vi "Write Observation Title.vi"(8 "error in (no error)":errorcluster, 10 "OBS_TITLE.Value":string, 11 "Save Image in":refnum<class "Save Image.lvclass">) -> (0 "error out":errorcluster, 3 "Save Image out":refnum<class "Save Image.lvclass">)   [LabVIEW 2018]
uses:
  Save Image.lvclass
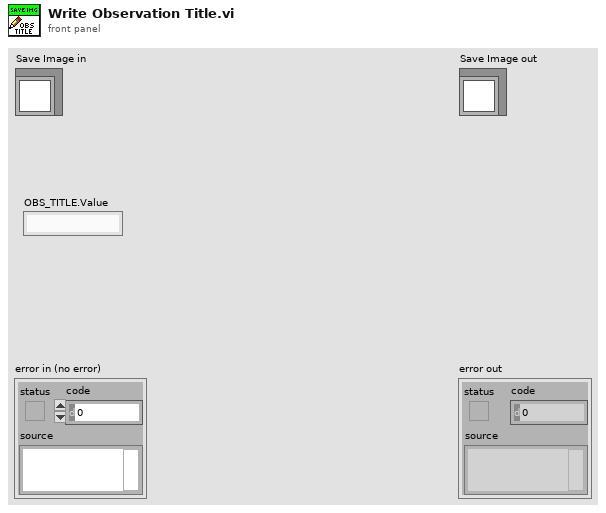
[diagram p1: front panel]
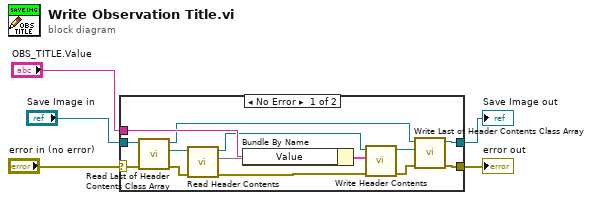
[diagram p0: block diagram]
diagram:
  n1 = case shown="No Error" "error in (no error)" {
    selector: "error in (no error)" -> [w11 w21]
    tunnel: [w14 w21] -> w4
    tunnel: [w13 w20] -> w2
    tunnel: "Save Image in" -> [w8 w20]
    tunnel: "OBS_TITLE.Value" -> [w19 _]
    frame No Error {
      n2 = call "Read Last of Header Contents Class Array.vi"("error in (no error)"=w11, "Save Image in"=w8) -> ("error out"=w10:errorcluster, "Simulated_Header.lvclass"=w9:refnum<class "Simulated_Header.lvclass">, "Save Image out"=w6:refnum<class "Save Image.lvclass">)  [unwired: 7 in]
      n3 = call "Read Header Contents.vi"("error in (no error)"=w10, "Header in"=w9) -> ("error out"=w15:errorcluster, 2:w17, "Header out"=w18:refnum<class "Simulated_Header.lvclass">)  [unwired: 7 in]
      n4 = Bundle By Name(cluster=w17, "Value"=w19) -> (w16:cluster{})
      n5 = call "Write Header Contents.vi"("error in (no error)"=w15, "Header Content"=w16, "Header in"=w18) -> ("error out"=w7:errorcluster, "Header out"=w12:refnum<class "Simulated_Header.lvclass">)  [unwired: 7 in]
      n6 = call "Write Last of Header Contents Class Array.vi"("error in (no error)"=w7, "Simulated_Header.lvclass"=w12, "Save Image in"=w6) -> ("error out"=w14:errorcluster, "Save Image out"=w13:refnum<class "Save Image.lvclass">)  [unwired: 7 in]
    }
    frame Error {
    }
  }
  "error out" <- w4
  "Save Image out" <- w2
